vi "Change Class Color.vi"() -> ()   [LabVIEW 2015]
uses:
  QControl Creation Script/QControl Creation.lvclass
  <vilib>/picture/picture.llb/imagedata.ctl
  <vilib>/Utility/miscctls.llb/LVPoint32TypeDef.ctl
  <vilib>/LabVIEW Icon API/API_User Layer Data.ctl
  <vilib>/LabVIEW Icon API/LabVIEW Icon API.lvlib
  <vilib>/LabVIEW Icon API/lv_icon/Classes/Icon/Icon.lvclass
  <vilib>/LabVIEW Icon API/API_Rectangle Dimension.ctl
  <vilib>/LabVIEW Icon API/API_Text.ctl
  <vilib>/LabVIEW Icon API/API_Text Colors.ctl
  <vilib>/LabVIEW Icon API/lv_icon/Controls/Alignment.ctl
  <vilib>/LabVIEW Icon API/API_Test Settings.ctl
  <vilib>/LabVIEW Icon API/lv_icon/Classes/Icon Framework/Icon Framework.lvclass
panel:
  in  "Class Path":path
  # "To update your QControl Class to the new standard color:\n\n1) Select the path to your class.\n2) Click Run."
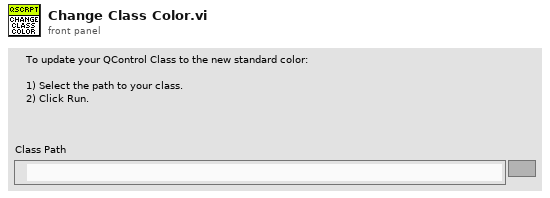
[diagram p1: front panel]
types:
  T1 = typedef "LabVIEW Icon API.lvlib/API_Test Settings.ctl" = cluster{"Font":string, "Alignment":T2, "Size":u8, "Center text":bool, "Capitalize text":bool, "Text color":T3}
  T2 = typedef "Alignment.ctl" = u16
  T3 = typedef "LabVIEW Icon API.lvlib/API_Text Colors.ctl" = cluster{"Line 1 color":u32, "Line 2 color":u32, "Line 3 color":u32, "Line 4 color":u32}
  T4 = typedef "LabVIEW Icon API.lvlib/API_Text.ctl" = cluster{"Line 1 text":string, "Line 2 text":string, "Line 3 text":string, "Line 4 text":string}
  T5 = typedef "LabVIEW Icon API.lvlib/API_Rectangle Dimension.ctl" = cluster{"Width":i16, "Height":i16}
  T6 = typedef "LabVIEW Icon API.lvlib/API_User Layer Data.ctl" = cluster{"Layer name":string, "Origin":T7, "Icon image data":T8}
  T7 = typedef "LVPoint32TypeDef.ctl" = cluster{"Horizontal":i32, "Vertical":i32}
  T8 = typedef "imagedata.ctl" = cluster{"image type":i32, "image depth":i32, "image":u8[], "mask":u8[], "colors":u32[], "Rectangle":cluster{"left":i16, "top":i16, "right":i16, "bottom":i16}}
  T9 = typedef "BodyText.ctl" = cluster{"Line 1 text":string, "Line 2 text":string, "Line 3 text":string, "Line 4 text":string, "Line 1 color":u32, "Line 2 color":u32, "Line 3 color":u32, "Line 4 color":u32, "Body Text Spec":cluster{"Font":T10, "Alignment":T2, "Size":u8}, "Center text vertically":bool, "Capitalize Text":bool}
  T10 = typedef "Font.ctl" = string
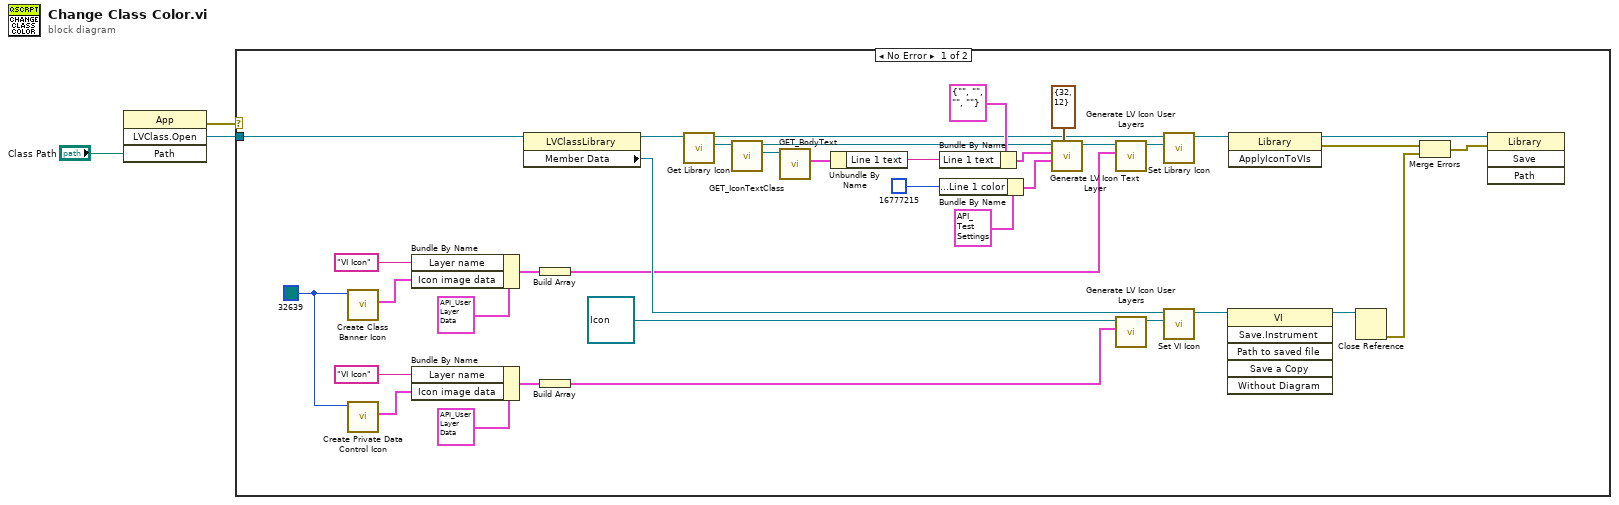
[diagram p0: block diagram]
diagram:
  n1 = invoke class="App" method="LVClass.Open"("Path"="Class Path") -> (error out=w2:errorcluster, "LVClass.Open"=w1:refnum<vi>)  [unwired: 3 in, 2 out]
  n2 = case shown="No Error" w2 {
    tunnel: w1 -> [w6 _]
    frame No Error {
      w40 = u32 32639
      n3 = call "Create Class Banner Icon.vi"("Theme Color"=w40) -> ("Icon Out"=w35:T8)  [unwired: 9 in, 1 out]
      n4 = call "Create Private Data Control Icon.vi"("Theme Color"=w40) -> ("Icon Out"=w39:T8)  [unwired: 9 in, 1 out]
      n5 = Bundle By Name(cluster=T6 {"Layer name"="", "Origin"={"Horizontal"=0, "Vertical"=0}, "Icon image data"={"image type"=0, "image depth"=0, "image"=[], "mask"=[], "colors"=[], "Rectangle"={"left"=0, "top"=0, "right"=0, "bottom"=0}}} ("User layer"), "Layer name"="VI Icon", "Icon image data"=w35) -> (w32:T6)
      n6 = Bundle By Name(cluster=T6 {"Layer name"="", "Origin"={"Horizontal"=0, "Vertical"=0}, "Icon image data"={"image type"=0, "image depth"=0, "image"=[], "mask"=[], "colors"=[], "Rectangle"={"left"=0, "top"=0, "right"=0, "bottom"=0}}} ("User layer"), "Layer name"="VI Icon", "Icon image data"=w39) -> (w38:T6)
      n7 = property class="LVClassLibrary"(reference=w6) -> (reference out=w7:refnum<vi>, "Member Data"=w10:refnum<vi>)  [unwired: 1 in, 1 out]
      n8 = Build Array(w32) -> (w5:T6[])
      n9 = Build Array(w38) -> (w4:T6[])
      n10 = call <vilib>:"Get Library Icon.vi"("Library Refnum in"=w7) -> ("Icon"=w20:refnum<class "Icon.lvclass">, "Library Refnum out"=w8:refnum<vi>)  [unwired: 8 in, 1 out]
      n11 = call-dynamic "GET_IconTextClass.vi"("Icon.lvclass in"=w20) -> ("Icon Framework.lvclass"=w21:refnum<class "Icon Framework.lvclass">, "Icon.lvclass out"=w23:refnum<class "Icon.lvclass">)  [unwired: 8 in, 1 out]
      n12 = call-dynamic "GET_BodyText.vi"("Icon Framework.lvclass in"=w21) -> ("Body Text"=w25:T9)  [unwired: 7 in, 3 out]
      n13 = Unbundle By Name(w25) -> ("Line 1 text"=w27:string)
      n14 = Bundle By Name(cluster=T4 {"Line 1 text"="", "Line 2 text"="", "Line 3 text"="", "Line 4 text"=""} ("Text"), "Line 1 text"=w27) -> (w28:T4)
      n15 = Bundle By Name(cluster=T1 {"Font"="Small Fonts", "Alignment"=1, "Size"=8, "Center text"=TRUE, "Capitalize text"=TRUE, "Text color"={"Line 1 color"=0, "Line 2 color"=0, "Line 3 color"=0, "Line 4 color"=0}} ("Text settings"), "Text color.Line 1 color"=u32 16777215) -> (w31:T1)
      n16 = call <vilib>:"Generate LV Icon Text Layer.vi"("Rectangle dimension (32,32)"=T5 {"Width"=32, "Height"=12}, "Text settings"=w31, "Text"=w28, "Icon in"=w23) -> ("Icon out"=w24:refnum<class "Icon.lvclass">)  [unwired: 6 in, 1 out]
      n17 = call <vilib>:"Generate LV Icon User Layers.vi"("User layers"=w5, "Icon in"=w24) -> ("Icon out"=w9:refnum<class "Icon.lvclass">)  [unwired: 8 in, 1 out]
      n18 = call <vilib>:"Generate LV Icon User Layers.vi"("User layers"=w4, "Icon in"=refnum<class "Icon.lvclass"> refnum ("Icon.lvclass in")) -> ("Icon out"=w12:refnum<class "Icon.lvclass">)  [unwired: 8 in, 1 out]
      n19 = call <vilib>:"Set Library Icon.vi"("Icon"=w9, "Library Refnum in"=w8) -> ("Library Refnum out"=w13:refnum<vi>)  [unwired: 8 in, 1 out]
      n20 = call <vilib>:"Set VI Icon.vi"("Icon"=w12, "VI Refnum in"=w10) -> ("VI Refnum out"=w14:refnum<vi>)  [unwired: 8 in, 1 out]
      n21 = invoke class="VI" method="Save.Instrument"(reference=w14) -> (reference out=w15:refnum<vi>)  [unwired: 5 in, 5 out]
      n22 = invoke class="Library" method="ApplyIconToVIs"(reference=w13) -> (reference out=w18:refnum<vi>, error out=w16:errorcluster)  [unwired: 2 in, 1 out]
      n23 = Close Reference(reference=w15) -> (error out=w17:errorcluster)  [unwired: 1 in]
      n24 = Merge Errors(w16, w17) -> (w19:errorcluster)
      n25 = invoke class="Library" method="Save"(reference=w18, error in=w19) -> ()  [unwired: 2 in, 4 out]
    }
    frame Error {
    }
  }
